vi "PH_Beckhoff.set Change Manager.vi"(0 "i ref in":refnum<vi>, 2 "Current Value Changes":T1, 3 "Old Value Changes":T1, 5 "error in":errorcluster) -> (14 "i ref out":refnum<vi>, 19 "error out":errorcluster)   [LabVIEW 2014, in "PH_Beckhoff.lvlib"]
doc: "This VI sets the attributes whether values have chnaged."
uses:
  PH_Beckhoff.lvlib
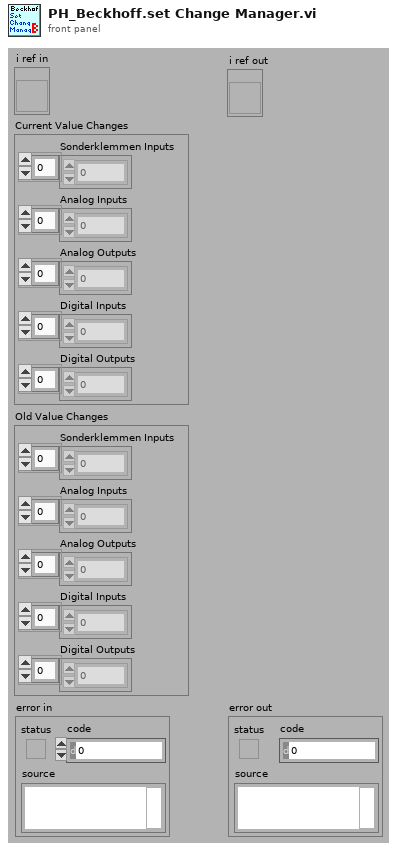
[diagram p1: front panel]
types:
  T1 = cluster{"Sonderklemmen Inputs":i32[], "Analog Inputs":i32[], "Analog Outputs":i32[], "Digital Inputs":i32[], "Digital Outputs":i32[]}
  T2 = typedef "PH_Beckhoff.lvlib/PH_Beckhoff.i attribute.ctl" = cluster{"GUI Refs":T3, "operation?":bool, "Default Prdc Interval":i32, "Connection":T4, "AMS Net ID":T5, "Klemmencluster: # of":T6, "Values":T7, "IP":string, "Description":string, "configured?":bool, "Change Manager":cluster{"Detemination wanted?":bool, "Values changed at":cluster{"Sonderklemmen Inputs":i32[], "Analog Inputs":i32[], "Analog Outputs":i32[], "Digital Inputs":i32[], "Digital Outputs":i32[]}}, "Difference to handle an analog input as change":u32}
  T3 = typedef "PH_Beckhoff.lvlib/PH_Beckhoff.GUI Refs.ctl" = cluster{"ADS Error":refnum<vi>, "Values":refnum<vi>, "configured?":refnum<vi>, "Connection":refnum<vi>, "IP":refnum<vi>, "Prdc Int [ms]":refnum<vi>}
  T4 = typedef "PH_Beckhoff.lvlib/PH_Beckhoff.Connectivity.ctl" = cluster{"DLL?":bool, "Port?":bool, "Client?":bool, "Ping?":bool, "unsuccessful Pings":u32}
  T5 = typedef "Beckhoff - Driver np.lvlib/Beckhoff Access.ctl" = cluster{"DLL path":path, "AMS Net ID":cluster{"1st # of IP":u8, "2nd # of IP":u8, "3rd # of IP":u8, "4th # of IP":u8, "In Port":u8, "Out Port":u8}}
  T6 = typedef "Beckhoff - Driver np.lvlib/Klemmendeclarer.ctl" = cluster{"Offset due to Sonderklemms":u32, "analog Inputs":u32, "analog Outputs":u32, "digital Input Bits":u32, "digital Output Bits":u32}
  T7 = typedef "PH_Beckhoff.lvlib/PH_Beckhoff.Values.ctl" = cluster{"Sonderklemmen Inputs":T8, "Analog Inputs":T9, "Analog Outputs":T11, "Digital Inputs":T12, "Digital Outputs":T13}
  T8 = typedef "PH_Beckhoff.lvlib/PH_Beckhoff.Sonderklemmen Inputs.ctl" = cluster{"Total Length":u32, "Name":string, "Value":u64, "Quality":bool, "Service ID":i32, "Offset":u32, "Length":u32}[]
  T9 = typedef "PH_Beckhoff.lvlib/PH_Beckhoff.Analog Inputs.ctl" = cluster{"Name":string, "Value":u32, "Quality":bool, "Service ID":i32, "Sca Type":T10}[]
  T10 = typedef "PH_Beckhoff.lvlib/PH_Beckhoff.Scaling Type.ctl" = enum16{"none", "0 ... 15 Bit -> 0 ... 5", "0 ... 15 Bit -> 0 ... 10", "0 ... 15 Bit -> 0 ... 25", "0 ... 15 Bit -> 4 ... 20", "0 ... 15 Bit -> 0 ... 1", "0 ... 15 Bit -> 0 ... 20000", "0 ... 15 Bit -> 0 ... 24000"}
  T11 = typedef "PH_Beckhoff.lvlib/PH_Beckhoff.Analog Outputs.ctl" = cluster{"Name":string, "Value":u32, "Quality":bool, "Wanted Value":u32, "Service ID":i32, "Sca Type":T10}[]
  T12 = typedef "PH_Beckhoff.lvlib/PH_Beckhoff.Digital Inputs.ctl" = cluster{"Name":string, "Value":bool, "Quality":bool, "Service ID":i32, "inverted?":bool}[]
  T13 = typedef "PH_Beckhoff.lvlib/PH_Beckhoff.Digital Outputs.ctl" = cluster{"Name":string, "Value":bool, "Quality":bool, "Wanted Value":bool, "Service ID":i32, "inverted?":bool}[]
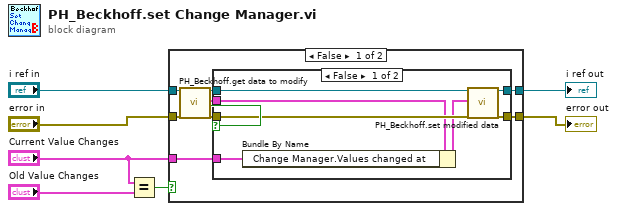
[diagram p0: block diagram]
diagram:
  n1 = Equal?(x="Current Value Changes", y="Old Value Changes") -> (x = y?=w7:bool)
  n2 = case shown="False" w7 {
    tunnel: "error in" -> [w16 w27]
    tunnel: [w10 w27] -> w6
    tunnel: [w11 w26] -> w4
    tunnel: "i ref in" -> [w9 w26]
    tunnel: "Current Value Changes" -> [w8 _]
    frame False {
      n3 = call "PH_Beckhoff.get data to modify.vi"("i ref in"=w9, "error in (no error)"=w16) -> ("i ref out"=w14:refnum<vi>, "i attribute"=w13:T2, "timed out"=w12:bool, "error out"=w15:errorcluster)  [unwired: 14 in]
      n4 = case shown="False" w12 {
        tunnel: w15 -> [w23 w24]
        tunnel: [w18 w24] -> w10
        tunnel: w14 -> [w22 w25]
        tunnel: [w19 w25] -> w11
        tunnel: w13 -> [w21 _]
        tunnel: w8 -> [w17 _]
        frame False {
          n5 = Bundle By Name(cluster=w21, "Change Manager.Values changed at"=w17) -> (w20:T2)
          n6 = call "PH_Beckhoff.set modified data.vi"("i ref in"=w22, "i attribute"=w20, "error in (no error)"=w23) -> ("i ref out"=w19:refnum<vi>, "error out"=w18:errorcluster)  [unwired: 15 in]
        }
        frame True {
        }
      }
    }
    frame True {
    }
  }
  "error out" <- w6
  "i ref out" <- w4
